vi "Extrae_SetVolt.vi"(10 "String":string="Set Voltage 4.2V at 20V/min, Sweep&meas") -> (1 "Array":string[](array[string]))   [LabVIEW 2017]
panel:
  # "Set Voltage 4.2V at 20V/min, Wait"
  # "Set Voltage 4.2V at 20V/min, Sweep&meas"
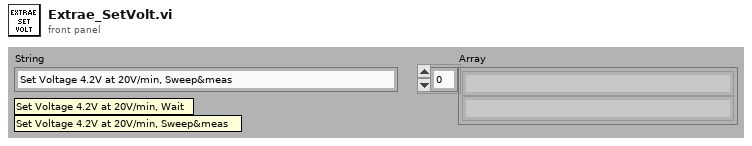
[diagram p1: front panel]
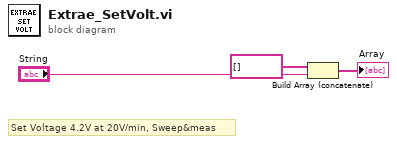
[diagram p0: block diagram]
diagram:
  # "Set Voltage 4.2V at 20V/min, Sweep&meas"
  n1 = Build Array (concatenate)(string[] [] ("Array I"), "String") -> (→"Array":string[])
